vi "Keithley24XX_settings_snap.vi"(8 "error in (no error)":errorcluster, 11 "VISA resource name":refnum<visa-resource-name>) -> (0 "error out":errorcluster, 2 "Keithley 24XX State":T1, 3 "VISA resource name 2":refnum<visa-resource-name>)   [LabVIEW 2018]
uses:
  <instrlib>/Keithley 24XX/Public/Data/Read (Single Point).vi
  <instrlib>/Keithley 24XX/Keithley 24XX.lvlib
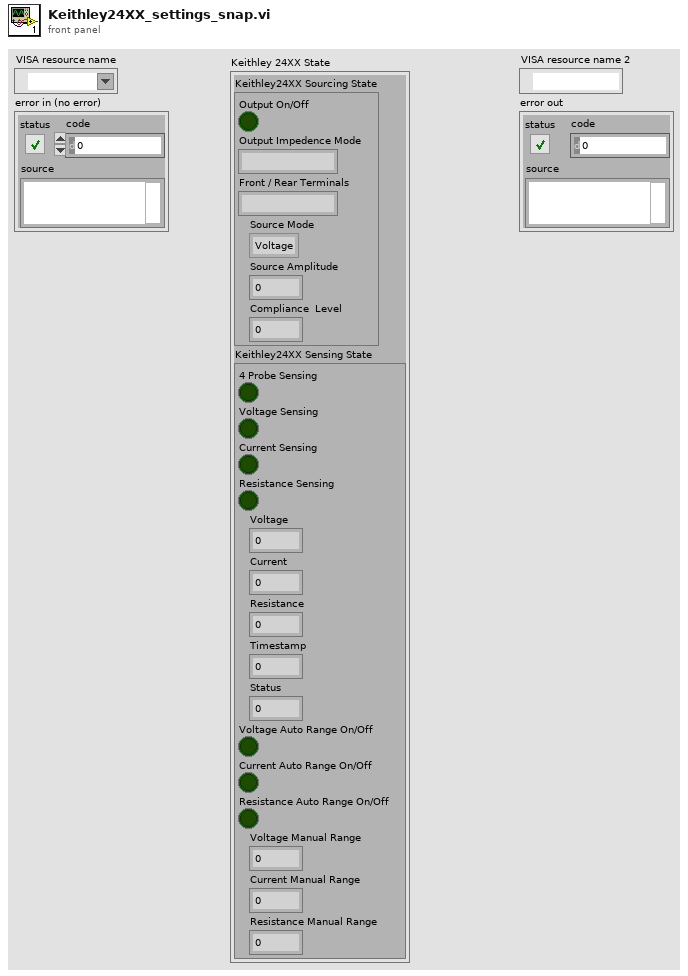
[diagram p1: front panel]
types:
  T1 = cluster{"Keithley24XX Sourcing State":cluster{"Output On/Off":bool, "Output Impedence Mode":string, "Front / Rear Terminals":string, "Source Mode":enum16{"Voltage", "Current"}, "Source Amplitude":dbl, "Compliance  Level":dbl}, "Keithley24XX Sensing State":cluster{"4 Probe Sensing":bool, "Voltage Sensing":bool, "Current Sensing":bool, "Resistance Sensing":bool, "Voltage":dbl, "Current":dbl, "Resistance":dbl, "Timestamp":dbl, "Status":dbl, "Voltage Auto Range On/Off":bool, "Current Auto Range On/Off":bool, "Resistance Auto Range On/Off":bool, "Voltage Manual Range":dbl, "Current Manual Range":dbl, "Resistance Manual Range":dbl}}
  T2 = cluster{"4 Probe Sensing":bool, "Voltage Sensing":bool, "Current Sensing":bool, "Resistance Sensing":bool, "Voltage":dbl, "Current":dbl, "Resistance":dbl, "Timestamp":dbl, "Status":dbl, "Voltage Auto Range On/Off":bool, "Current Auto Range On/Off":bool, "Resistance Auto Range On/Off":bool, "Voltage Manual Range":dbl, "Current Manual Range":dbl, "Resistance Manual Range":dbl}
  T3 = cluster{"Output On/Off":bool, "Output Impedence Mode":string, "Front / Rear Terminals":string, "Source Mode":enum16{"Voltage", "Current"}, "Source Amplitude":dbl, "Compliance  Level":dbl}
  T4 = cluster{"VISA resource name":refnum<visa-resource-name>, "error out":errorcluster}
  T5 = cluster{"VISA resource name out":refnum<visa-resource-name>, "error out":errorcluster}
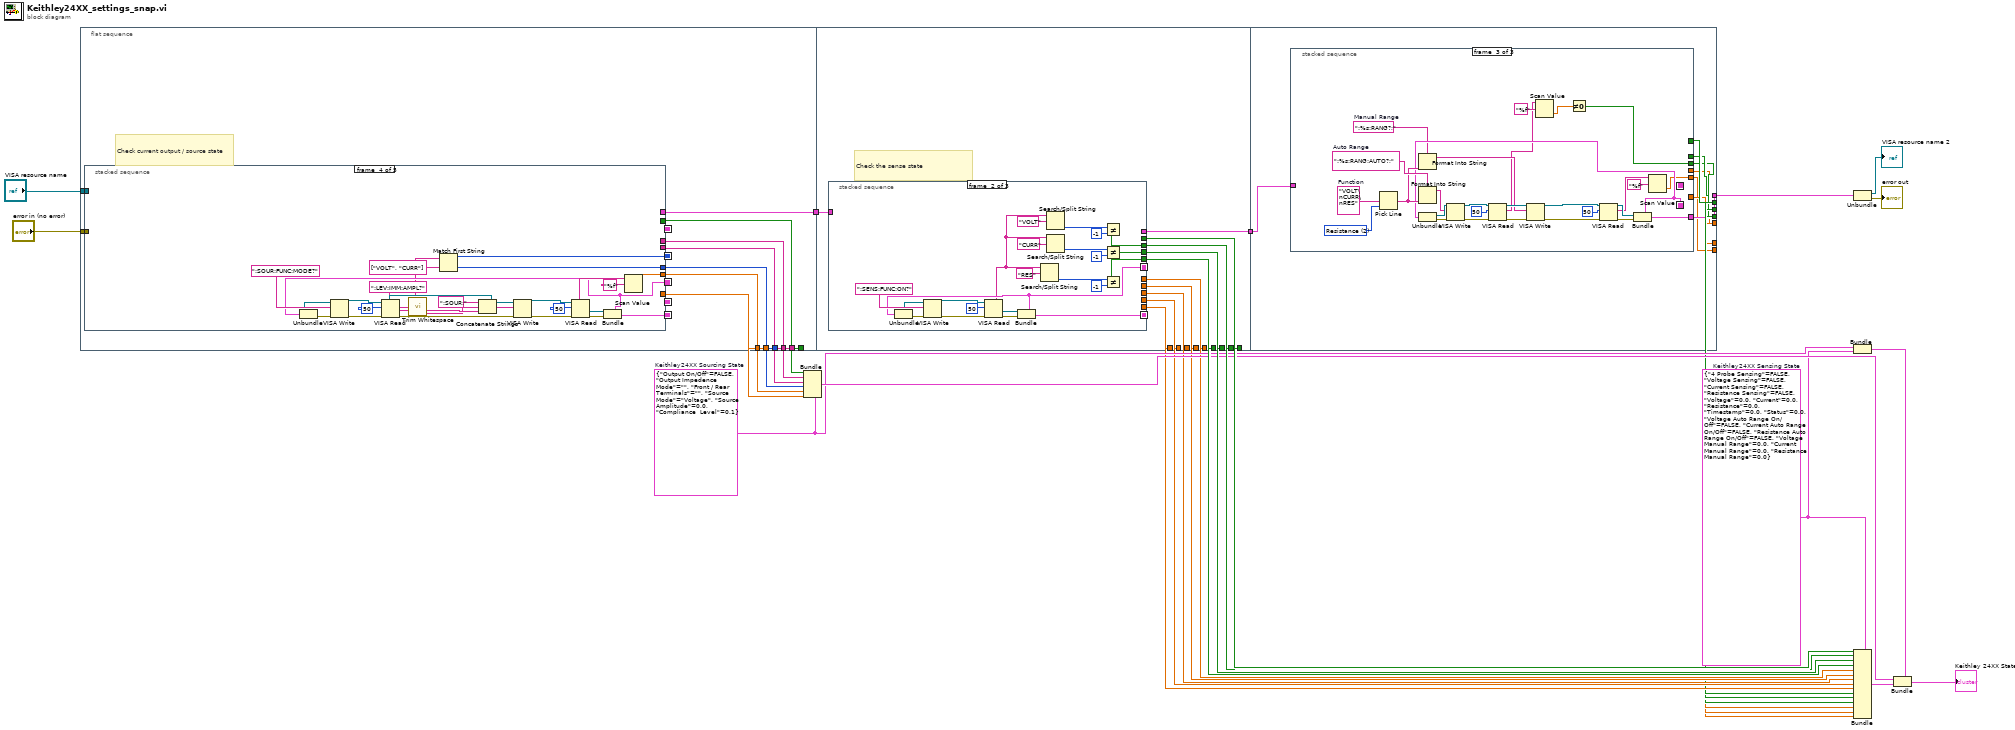
[diagram p0: block diagram]
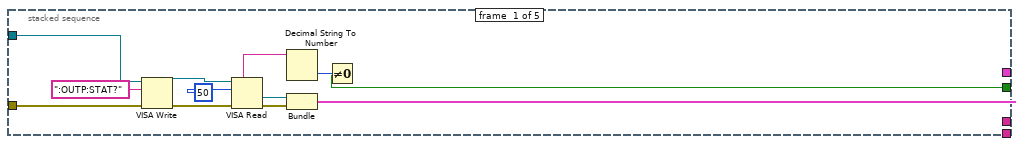
[diagram p2: hidden frame]
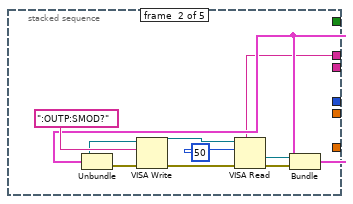
[diagram p3: hidden frame]
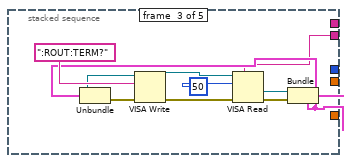
[diagram p4: hidden frame]
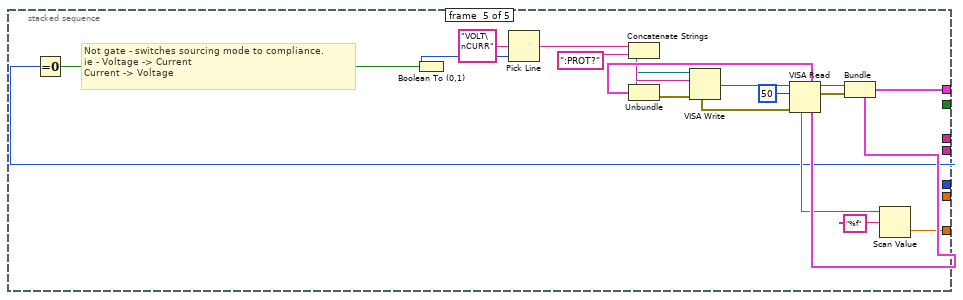
[diagram p5: hidden frame]
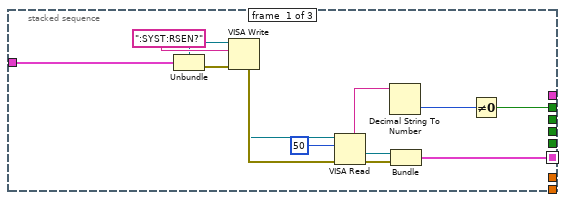
[diagram p6: hidden frame]
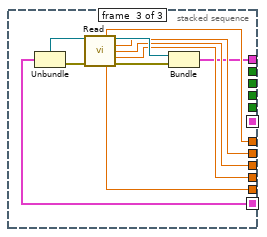
[diagram p7: hidden frame]
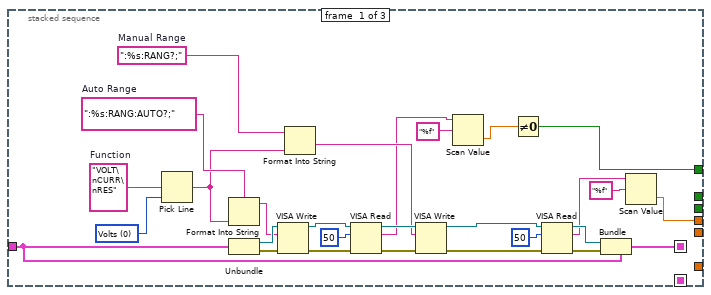
[diagram p8: hidden frame]
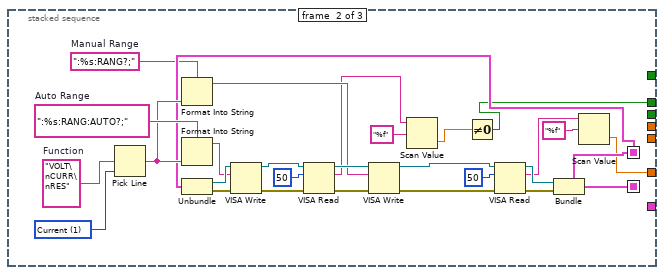
[diagram p9: hidden frame]
diagram:
  w15 = T2 {"4 Probe Sensing"=FALSE, "Voltage Sensing"=FALSE, "Current Sensing"=FALSE, "Resistance Sensing"=FALSE, "Voltage"=0.0, "Current"=0.0, "Resistance"=0.0, "Timestamp"=0.0, "Status"=0.0, "Voltage Auto Range On/Off"=FALSE, "Current Auto Range On/Off"=FALSE, "Resistance Auto Range On/Off"=FALSE, "Voltage Manual Range"=0.0, "Current Manual Range"=0.0, "Resistance Manual Range"=0.0}  # Keithley24XX Sensing State
  w16 = T3 {"Output On/Off"=FALSE, "Output Impedence Mode"="", "Front / Rear Terminals"="", "Source Mode"=enum."Voltage", "Source Amplitude"=0.0, "Compliance  Level"=0.1}  # Keithley24XX Sourcing State
  n1 = flat-sequence {
    tunnel: "VISA resource name" -> [w43]
    tunnel: "error in (no error)" -> [w42]
    tunnel: [w41] -> w28
    tunnel: [w40] -> w27
    tunnel: [w39] -> w26
    tunnel: [w38] -> w25
    tunnel: [w37] -> w24
    tunnel: [w36] -> w23
    tunnel: [w35] -> w13
    tunnel: [w132] -> w32
    tunnel: [w131] -> w22
    tunnel: [w130] -> w21
    tunnel: [w129] -> w20
    tunnel: [w128] -> w19
    tunnel: w13 -> [w127]
    tunnel: [w126] -> w12
    tunnel: [w125] -> w11
    tunnel: [w124] -> w10
    tunnel: [w123] -> w9
    tunnel: [w122] -> w8
    tunnel: w32 -> [w186]
    tunnel: [w187] -> w31
    tunnel: [w185] -> w7
    tunnel: [w184] -> w6
    tunnel: [w183] -> w5
    tunnel: [w182] -> w4
    tunnel: [w181] -> w3
    tunnel: [w180] -> w2
    frame #0 {
      # "Check current output / source state"
      n2 = stacked-sequence {
        seq-local: [w45 _ _ _ _] -> [_ w58 _ _ _]
        seq-local: [_ w57 _ _ _] -> [_ _ w73 _ _]
        seq-local: [_ _ w68 _ _] -> [_ _ _ w88 _]
        seq-local: [_ _ _ w81 _] -> [_ _ _ _ w121]
        seq-local: [_ _ _ w78 _] -> [_ _ _ _ w105]
        tunnel: w43 -> [w49 _ _ _ _]
        tunnel: w42 -> [w48 _ _ _ _]
        tunnel: [w44 _ _ _ _] -> w41
        tunnel: [_ w56 _ _ _] -> w40
        tunnel: [_ _ w67 _ _] -> w39
        tunnel: [_ _ _ w82 _] -> w38
        tunnel: [_ _ _ w78 _] -> w37
        tunnel: [_ _ _ _ w107] -> w36
        tunnel: [_ _ _ _ w106] -> w35
        frame #0 {
          n3 = VISA Write(VISA resource name=w49, write buffer=":OUTP:STAT?", error in (no error)=w48) -> (VISA resource name out=w52:refnum<visa-resource-name>, error out=w55:errorcluster)  [unwired: 1 out]
          n4 = VISA Read(VISA resource name=w52, byte count=u32 50, error in (no error)=w55) -> (VISA resource name out=w47:refnum<visa-resource-name>, read buffer=w51:string, error out=w46:errorcluster)  [unwired: 1 out]
          n5 = Decimal String To Number(string=w51) -> (number=w50:i32)  [unwired: 2 in, 1 out]
          n6 = Bundle("VISA resource name"=w47, "error out"=w46) -> (w45:T4)  [unwired: 1 in]
          n7 = Not Equal To 0?(x=w50) -> (x != 0?=w44:bool)
        }
        frame #1 {
          n8 = Unbundle(w58) -> ("VISA resource name"=w62:refnum<visa-resource-name>, "error out"=w61:errorcluster)
          n9 = VISA Write(VISA resource name=w62, write buffer=":OUTP:SMOD?", error in (no error)=w61) -> (VISA resource name out=w63:refnum<visa-resource-name>, error out=w66:errorcluster)  [unwired: 1 out]
          n10 = VISA Read(VISA resource name=w63, byte count=u32 50, error in (no error)=w66) -> (VISA resource name out=w59:refnum<visa-resource-name>, read buffer=w56:string, error out=w60:errorcluster)  [unwired: 1 out]
          n11 = Bundle(cluster=w58, "VISA resource name"=w59, "error out"=w60) -> (w57:T4)
        }
        frame #2 {
          n12 = Unbundle(w73) -> ("VISA resource name"=w72:refnum<visa-resource-name>, "error out"=w71:errorcluster)
          n13 = VISA Write(VISA resource name=w72, write buffer=":ROUT:TERM?", error in (no error)=w71) -> (VISA resource name out=w74:refnum<visa-resource-name>, error out=w77:errorcluster)  [unwired: 1 out]
          n14 = VISA Read(VISA resource name=w74, byte count=u32 50, error in (no error)=w77) -> (VISA resource name out=w70:refnum<visa-resource-name>, read buffer=w67:string, error out=w69:errorcluster)  [unwired: 1 out]
          n15 = Bundle(cluster=w73, "VISA resource name"=w70, "error out"=w69) -> (w68:T4)
        }
        frame #3 {
          n16 = Unbundle(w88) -> ("VISA resource name"=w87:refnum<visa-resource-name>, "error out"=w86:errorcluster)
          n17 = VISA Write(VISA resource name=w87, write buffer=":SOUR:FUNC:MODE?", error in (no error)=w86) -> (VISA resource name out=w99:refnum<visa-resource-name>, error out=w102:errorcluster)  [unwired: 1 out]
          n18 = VISA Read(VISA resource name=w99, byte count=u32 50, error in (no error)=w102) -> (VISA resource name out=w94:refnum<visa-resource-name>, read buffer=w83:string, error out=w95:errorcluster)  [unwired: 1 out]
          n19 = call <vilib>:"Trim Whitespace.vi"("string"=w83) -> ("trimmed string"=w79:string)  [unwired: 1 in]
          n20 = Match First String(2:string[] ["VOLT", "CURR"] ("string array"), 3:w79) -> (0:w78:i32)  [unwired: 1 out]
          n21 = Concatenate Strings(":SOUR:" ("string"), w79, ":LEV:IMM:AMPL?" ("string")) -> (w91:string)
          n22 = VISA Write(VISA resource name=w94, write buffer=w91, error in (no error)=w95) -> (VISA resource name out=w96:refnum<visa-resource-name>, error out=w98:errorcluster)  [unwired: 1 out]
          n23 = VISA Read(VISA resource name=w96, byte count=u32 50, error in (no error)=w98) -> (VISA resource name out=w85:refnum<visa-resource-name>, read buffer=w89:string, error out=w84:errorcluster)  [unwired: 1 out]
          n24 = Bundle(cluster=w88, "VISA resource name"=w85, "error out"=w84) -> (w81:T4)
          n25 = Scan Value(string=w89, format string="%f") -> (value=w82:dbl)  [unwired: 1 in, 1 out]
        }
        frame #4 {
          # "Not gate - switches sourcing mode to compliance. \nie - Voltage -> Current\nCurrent -> Voltage"
          n26 = Equal To 0?(x=w105) -> (x = 0?=w104:bool)
          n27 = Boolean To (0,1)(Boolean=w104) -> (0, 1=w103:i16)
          n28 = Pick Line(multi-line string="VOLT\nCURR", line index=w103) -> (output string=w115:string)  [unwired: 1 in]
          n29 = Concatenate Strings(w115, ":PROT?" ("string")) -> (w116:string)
          n30 = Unbundle(w121) -> ("VISA resource name"=w113:refnum<visa-resource-name>, "error out"=w112:errorcluster)
          n31 = VISA Write(VISA resource name=w113, write buffer=w116, error in (no error)=w112) -> (VISA resource name out=w117:refnum<visa-resource-name>, error out=w119:errorcluster)  [unwired: 1 out]
          n32 = VISA Read(VISA resource name=w117, byte count=u32 50, error in (no error)=w119) -> (VISA resource name out=w111:refnum<visa-resource-name>, read buffer=w108:string, error out=w110:errorcluster)  [unwired: 1 out]
          n33 = Bundle(cluster=w121, "VISA resource name"=w111, "error out"=w110) -> (w106:T4)
          n34 = Scan Value(string=w108, format string="%f") -> (value=w107:dbl)  [unwired: 1 in, 1 out]
        }
      }
    }
    frame #1 {
      # "Check the sense state"
      n35 = stacked-sequence {
        seq-local: [w137 _ _] -> [_ w164 _]
        seq-local: [_ w146 _] -> [_ _ w179]
        tunnel: [_ _ w169] -> w132
        tunnel: [w136 _ _] -> w131
        tunnel: [_ w149 _] -> w130
        tunnel: [_ w148 _] -> w129
        tunnel: [_ w147 _] -> w128
        tunnel: w127 -> [w135 _ _]
        tunnel: [_ _ w174] -> w126
        tunnel: [_ _ w173] -> w125
        tunnel: [_ _ w172] -> w124
        tunnel: [_ _ w171] -> w123
        tunnel: [_ _ w170] -> w122
        frame #0 {
          n36 = Unbundle(w135) -> ("VISA resource name"=w134:refnum<visa-resource-name>, "error out"=w133:errorcluster)
          n37 = VISA Write(VISA resource name=w134, write buffer=":SYST:RSEN?", error in (no error)=w133) -> (VISA resource name out=w142:refnum<visa-resource-name>, error out=w145:errorcluster)  [unwired: 1 out]
          n38 = VISA Read(VISA resource name=w142, byte count=u32 50, error in (no error)=w145) -> (VISA resource name out=w139:refnum<visa-resource-name>, read buffer=w141:string, error out=w138:errorcluster)  [unwired: 1 out]
          n39 = Decimal String To Number(string=w141) -> (number=w140:i32)  [unwired: 2 in, 1 out]
          n40 = Bundle("VISA resource name"=w139, "error out"=w138) -> (w137:T4)  [unwired: 1 in]
          n41 = Not Equal To 0?(x=w140) -> (x != 0?=w136:bool)
        }
        frame #1 {
          n42 = Unbundle(w164) -> ("VISA resource name"=w163:refnum<visa-resource-name>, "error out"=w162:errorcluster)
          n43 = VISA Write(VISA resource name=w163, write buffer=":SENS:FUNC:ON?", error in (no error)=w162) -> (VISA resource name out=w165:refnum<visa-resource-name>, error out=w168:errorcluster)  [unwired: 1 out]
          n44 = VISA Read(VISA resource name=w165, byte count=u32 50, error in (no error)=w168) -> (VISA resource name out=w161:refnum<visa-resource-name>, read buffer=w156:string, error out=w160:errorcluster)  [unwired: 1 out]
          n45 = Bundle(cluster=w164, "VISA resource name"=w161, "error out"=w160) -> (w146:T4)
          n46 = Search/Split String(string=w156, search string/char (-)="RES" ("true string")) -> (offset of match=w150:i32)  [unwired: 1 in, 2 out]
          n47 = Search/Split String(string=w156, search string/char (-)="VOLT" ("true string")) -> (offset of match=w155:i32)  [unwired: 1 in, 2 out]
          n48 = Search/Split String(string=w156, search string/char (-)="CURR" ("true string")) -> (offset of match=w152:i32)  [unwired: 1 in, 2 out]
          n49 = Not Equal?(x=w155, y=-1) -> (x != y?=w149:bool)
          n50 = Not Equal?(x=w152, y=-1) -> (x != y?=w148:bool)
          n51 = Not Equal?(x=w150, y=-1) -> (x != y?=w147:bool)
        }
        frame #2 {
          n52 = Unbundle(w179) -> ("VISA resource name"=w178:refnum<visa-resource-name>, "error out"=w177:errorcluster)
          n53 = call-poly <instrlib>:"Read.vi"("VISA resource name"=w178, "error in (no error)"=w177) -> ("Voltage"=w170:sgl, "VISA resource name out"=w175:refnum<visa-resource-name>, "Current"=w171:sgl, "Resistance"=w172:sgl, "Timestamp"=w173:sgl, "Status"=w174:sgl, "error out"=w176:errorcluster)  [unwired: 7 in]
          n54 = Bundle("VISA resource name out"=w175, "error out"=w176) -> (w169:T5)  [unwired: 1 in]
        }
      }
    }
    frame #2 {
      n55 = stacked-sequence {
        seq-local: [w195 _ _] -> [_ w225 _]
        seq-local: [_ w224 _] -> [_ _ w253]
        tunnel: w186 -> [w211 _ _]
        tunnel: [_ _ w252] -> w187
        tunnel: [w188 _ _] -> w185
        tunnel: [_ w216 _] -> w184
        tunnel: [_ _ w244] -> w183
        tunnel: [w192 _ _] -> w182
        tunnel: [_ w221 _] -> w181
        tunnel: [_ _ w249] -> w180
        frame #0 {
          w214 = u16 0 items=["Volts", "Current", "Resistance"] ("Function (0: Volts)")
          w210 = ":%s:RANG?;"  # Manual Range
          w213 = ":%s:RANG:AUTO?;"  # Auto Range
          w215 = "VOLT\nCURR\nRES"  # Function
          n56 = Pick Line(multi-line string=w215, line index=w214) -> (output string=w212:string)  [unwired: 1 in]
          n57 = Format Into String(format string=w213, w212) -> (resulting string=w199:string)  [unwired: 2 in, 1 out]
          n58 = Unbundle(w211) -> ("VISA resource name out"=w201:refnum<visa-resource-name>, "error out"=w200:errorcluster)
          n59 = VISA Write(VISA resource name=w201, write buffer=w199, error in (no error)=w200) -> (VISA resource name out=w207:refnum<visa-resource-name>, error out=w209:errorcluster)  [unwired: 1 out]
          n60 = Format Into String(format string=w210, w212) -> (resulting string=w198:string)  [unwired: 2 in, 1 out]
          n61 = VISA Read(VISA resource name=w207, byte count=u32 50, error in (no error)=w209) -> (VISA resource name out=w203:refnum<visa-resource-name>, read buffer=w190:string, error out=w202:errorcluster)  [unwired: 1 out]
          n62 = VISA Write(VISA resource name=w203, write buffer=w198, error in (no error)=w202) -> (VISA resource name out=w204:refnum<visa-resource-name>, error out=w206:errorcluster)  [unwired: 1 out]
          n63 = Scan Value(string=w190, format string="%f") -> (value=w189:dbl)  [unwired: 1 in, 1 out]
          n64 = Not Equal To 0?(x=w189) -> (x != 0?=w188:bool)
          n65 = VISA Read(VISA resource name=w204, byte count=u32 50, error in (no error)=w206) -> (VISA resource name out=w196:refnum<visa-resource-name>, read buffer=w193:string, error out=w197:errorcluster)  [unwired: 1 out]
          n66 = Bundle(cluster=w211, "VISA resource name out"=w196, "error out"=w197) -> (w195:T5)
          n67 = Scan Value(string=w193, format string="%f") -> (value=w192:dbl)  [unwired: 1 in, 1 out]
        }
        frame #1 {
          w220 = ":%s:RANG?;"  # Manual Range
          w242 = u16 1 items=["Volts", "Current", "Resistance"] ("Function (0: Volts) 2")
          w241 = ":%s:RANG:AUTO?;"  # Auto Range
          w243 = "VOLT\nCURR\nRES"  # Function
          n68 = Pick Line(multi-line string=w243, line index=w242) -> (output string=w240:string)  [unwired: 1 in]
          n69 = Format Into String(format string=w220, w240) -> (resulting string=w228:string)  [unwired: 2 in, 1 out]
          n70 = Format Into String(format string=w241, w240) -> (resulting string=w229:string)  [unwired: 2 in, 1 out]
          n71 = Unbundle(w225) -> ("VISA resource name out"=w231:refnum<visa-resource-name>, "error out"=w230:errorcluster)
          n72 = VISA Write(VISA resource name=w231, write buffer=w229, error in (no error)=w230) -> (VISA resource name out=w237:refnum<visa-resource-name>, error out=w239:errorcluster)  [unwired: 1 out]
          n73 = VISA Read(VISA resource name=w237, byte count=u32 50, error in (no error)=w239) -> (VISA resource name out=w233:refnum<visa-resource-name>, read buffer=w217:string, error out=w232:errorcluster)  [unwired: 1 out]
          n74 = VISA Write(VISA resource name=w233, write buffer=w228, error in (no error)=w232) -> (VISA resource name out=w234:refnum<visa-resource-name>, error out=w236:errorcluster)  [unwired: 1 out]
          n75 = Scan Value(string=w217, format string="%f") -> (value=w219:dbl)  [unwired: 1 in, 1 out]
          n76 = Not Equal To 0?(x=w219) -> (x != 0?=w216:bool)
          n77 = VISA Read(VISA resource name=w234, byte count=u32 50, error in (no error)=w236) -> (VISA resource name out=w226:refnum<visa-resource-name>, read buffer=w222:string, error out=w227:errorcluster)  [unwired: 1 out]
          n78 = Bundle(cluster=w225, "VISA resource name out"=w226, "error out"=w227) -> (w224:T5)
          n79 = Scan Value(string=w222, format string="%f") -> (value=w221:dbl)  [unwired: 1 in, 1 out]
        }
        frame #2 {
          w248 = ":%s:RANG?;"  # Manual Range
          w270 = u16 2 items=["Volts", "Current", "Resistance"] ("Function (0: Volts) 3")
          w269 = ":%s:RANG:AUTO?;"  # Auto Range
          w271 = "VOLT\nCURR\nRES"  # Function
          n80 = Pick Line(multi-line string=w271, line index=w270) -> (output string=w268:string)  [unwired: 1 in]
          n81 = Format Into String(format string=w248, w268) -> (resulting string=w256:string)  [unwired: 2 in, 1 out]
          n82 = Format Into String(format string=w269, w268) -> (resulting string=w257:string)  [unwired: 2 in, 1 out]
          n83 = Unbundle(w253) -> ("VISA resource name out"=w259:refnum<visa-resource-name>, "error out"=w258:errorcluster)
          n84 = VISA Write(VISA resource name=w259, write buffer=w257, error in (no error)=w258) -> (VISA resource name out=w265:refnum<visa-resource-name>, error out=w267:errorcluster)  [unwired: 1 out]
          n85 = VISA Read(VISA resource name=w265, byte count=u32 50, error in (no error)=w267) -> (VISA resource name out=w261:refnum<visa-resource-name>, read buffer=w245:string, error out=w260:errorcluster)  [unwired: 1 out]
          n86 = VISA Write(VISA resource name=w261, write buffer=w256, error in (no error)=w260) -> (VISA resource name out=w262:refnum<visa-resource-name>, error out=w264:errorcluster)  [unwired: 1 out]
          n87 = Scan Value(string=w245, format string="%f") -> (value=w247:dbl)  [unwired: 1 in, 1 out]
          n88 = Not Equal To 0?(x=w247) -> (x != 0?=w244:bool)
          n89 = VISA Read(VISA resource name=w262, byte count=u32 50, error in (no error)=w264) -> (VISA resource name out=w254:refnum<visa-resource-name>, read buffer=w250:string, error out=w255:errorcluster)  [unwired: 1 out]
          n90 = Bundle(cluster=w253, "VISA resource name out"=w254, "error out"=w255) -> (w252:T5)
          n91 = Scan Value(string=w250, format string="%f") -> (value=w249:dbl)  [unwired: 1 in, 1 out]
        }
      }
    }
  }
  n92 = Bundle(cluster=w16, "Output On/Off"=w28, "Output Impedence Mode"=w27, "Front / Rear Terminals"=w26, "Source Mode"=w24, "Source Amplitude"=w25, "Compliance  Level"=w23) -> (w18:T3)
  n93 = Unbundle(w31) -> ("VISA resource name out"=→"VISA resource name 2":refnum<visa-resource-name>, "error out"=→"error out":errorcluster)
  n94 = Bundle("Keithley24XX Sourcing State"=w16, "Keithley24XX Sensing State"=w15) -> (w14:T1)  [unwired: 1 in]
  n95 = Bundle(cluster=w15, "4 Probe Sensing"=w22, "Voltage Sensing"=w21, "Current Sensing"=w20, "Resistance Sensing"=w19, "Voltage"=w8, "Current"=w9, "Resistance"=w10, "Timestamp"=w11, "Status"=w12, "Voltage Auto Range On/Off"=w7, "Current Auto Range On/Off"=w6, "Resistance Auto Range On/Off"=w5, "Voltage Manual Range"=w4, "Current Manual Range"=w3, "Resistance Manual Range"=w2) -> (w17:T2)
  n96 = Bundle(cluster=w14, "Keithley24XX Sourcing State"=w18, "Keithley24XX Sensing State"=w17) -> (→"Keithley 24XX State":T1)
